vi "Get Oscillator Freq.vi"(5 "error in (no error)":errorcluster, 6 "Reference Clock":dbl, 7 "Array 3":string[](array[string])) -> (0 "Reference Clock Multiplier":dbl[](array[numeric]), 1 "error out":errorcluster, 2 "Oscillator Freqs":dbl[](array[numeric]), 3 "Tuning Word":string[](array[string]), 4 "Scaling Factor":dbl[](array[numeric]))   [LabVIEW 2018]
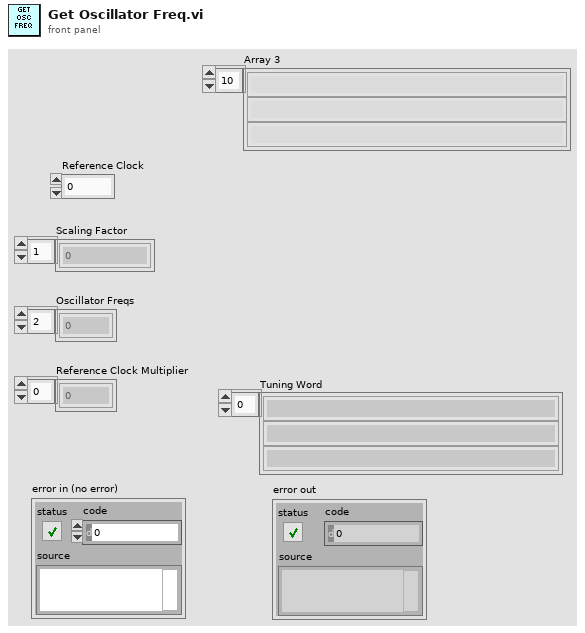
[diagram p1: front panel]
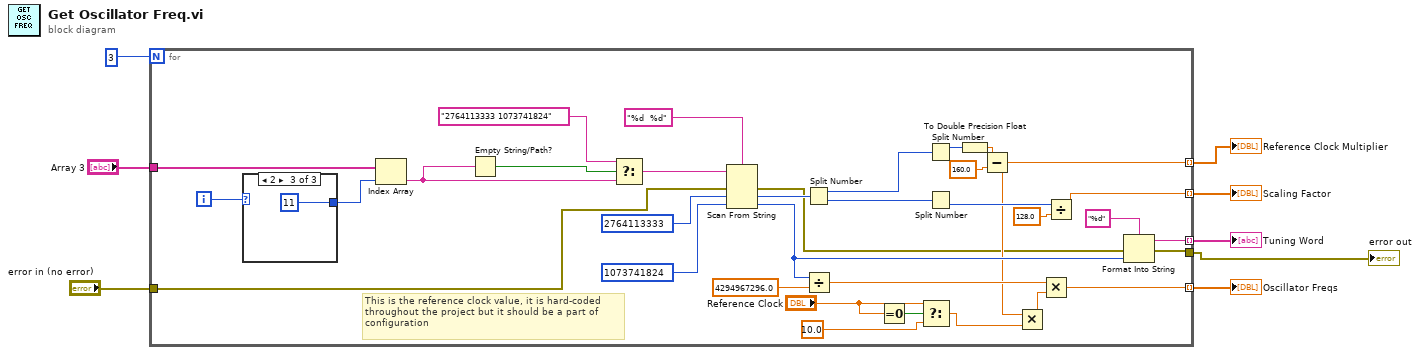
[diagram p0: block diagram]
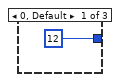
[diagram p2: hidden frame]
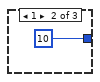
[diagram p3: hidden frame]
diagram:
  n1 = for {
    N: 3 -> [_]
    tunnel: "Array 3" -> [w41]
    tunnel: [w30] -> w8 mode=indexing
    tunnel: [w27] -> w7 mode=indexing
    tunnel: [w23] -> w4 mode=indexing
    tunnel: [w17] -> w3 mode=indexing
    tunnel: "error in (no error)" -> [w11]
    tunnel: [w9] -> w1
    i -> [w42]
    # "This is the reference clock value, it is hard-coded \nthroughout the project but it should be a part of\nconfiguration"
    n2 = case shown="2" w42 {
      tunnel: [12 ("y") 10 ("y") 11 ("y")] -> w40
      frame 0, Default {
      }
      frame 1 {
      }
      frame 2 {
      }
    }
    n3 = Index Array(array=w41, index=w40) -> (element=w35:string)
    n4 = Empty String/Path?(string/path=w35) -> (empty?=w38:bool)
    n5 = Select(t="2764113333 1073741824", s=w38, f=w35) -> (s? t:f=w36:string)
    n6 = Scan From String(format string="%d  %d", input string=w36, error in=w11, default 1=u32 2764113333 ("default value 1"), default 2=u32 1073741824 ("default value 1")) -> (error out=w10:errorcluster, output 1=w18:u32, output 2=w28:u32)  [unwired: 1 in, 2 out]
    n7 = Split Number(x=w18) -> (hi(x)=w22:u16, lo(x)=w26:u16)
    n8 = Divide(x=w28, y=4294967296.0) -> (x/y=w31:dbl)
    n9 = Equal To 0?(x="Reference Clock") -> (x = 0?=w13:bool)
    n10 = Select(t="Reference Clock", s=w13, f=10.0 ("y")) -> (s? t:f=w12:dbl)
    n11 = Split Number(x=w22) -> (hi(x)=w21:u8)  [unwired: 1 out]
    n12 = Split Number(x=w26) -> (lo(x)=w25:u8)  [unwired: 1 out]
    n13 = To Double Precision Float(number=w21) -> (double precision float=w20:dbl)
    n14 = Subtract(x=w20, y=160.0) -> (x-y=w17:dbl)
    n15 = Multiply(x=w17, y=w12) -> (x*y=w16:dbl)
    n16 = Multiply(x=w31, y=w16) -> (x*y=w30:dbl)
    n17 = Divide(x=w25, y=128.0) -> (x/y=w23:dbl)
    n18 = Format Into String(format string="%d", error in=w10, w28) -> (resulting string=w27:string, error out=w9:errorcluster)  [unwired: 1 in]
  }
  "Oscillator Freqs" <- w8
  "Tuning Word" <- w7
  "Scaling Factor" <- w4
  "Reference Clock Multiplier" <- w3
  "error out" <- w1
